vi "Read Items.vi"(8 "error in (no error)":errorcluster, 10 "After (all)":timestamp, 11 "Feed.lvclass in":refnum<class "Feed.lvclass">) -> (0 "error out":errorcluster, 2 "Items":refnum<class "FeedItem.lvclass">[](array[class]), 3 "Feed.lvclass out":refnum<class "Feed.lvclass">)   [LabVIEW 2020, in "Feed.lvclass"]
uses:
  <vilib>/NI_RSS/Feed/Feed.lvclass
  <vilib>/NI_RSS/FeedItem/FeedItem.lvclass
  <vilib>/NI_RSS/Feed/Feed.lvclass/Feed.ctl
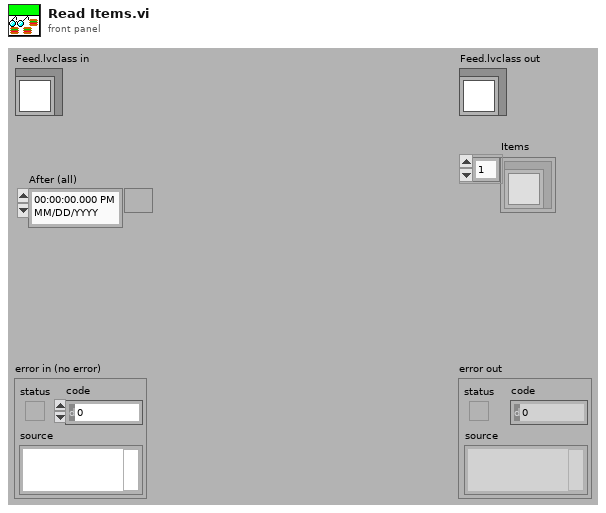
[diagram p1: front panel]
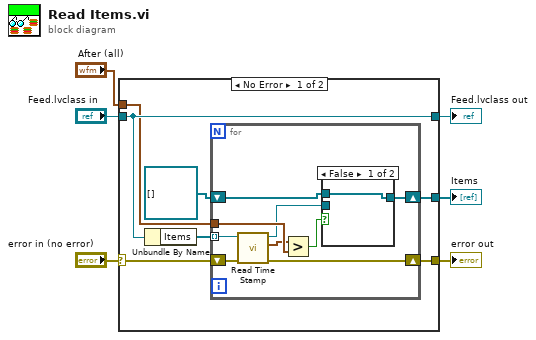
[diagram p0: block diagram]
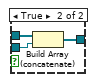
[diagram p2: hidden frame]
diagram:
  n1 = case shown="No Error" "error in (no error)" {
    selector: "error in (no error)" -> [w10 w27]
    tunnel: [w9 w27] -> w5
    tunnel: [w13 w28] -> w3
    tunnel: "Feed.lvclass in" -> [w13 w28]
    tunnel: [w7 _] -> w2
    tunnel: "After (all)" -> [w11 _]
    frame No Error {
      n2 = Unbundle By Name(w13) -> ("Items"=w12:refnum<class "FeedItem.lvclass">[])
      n3 = for {
        tunnel: w12 -> [w21] mode=indexing
        shift-right: [w14] -> w7
        shift-left: refnum<class "FeedItem.lvclass">[] [] -> [w16]
        tunnel: w11 -> [w22]
        shift-right: [w18] -> w9
        shift-left: w10 -> [w19]
        n4 = call-dynamic "Read Time Stamp.vi"("error in (no error)"=w19, "FeedItem.lvclass in"=w21) -> ("error out"=w18:errorcluster, "Time Stamp"=w20:timestamp, "FeedItem.lvclass out"=w15:refnum<class "FeedItem.lvclass">)  [unwired: 7 out]
        n5 = Greater?(x=w20, y=w22) -> (0:w17:bool)
        n6 = case shown="False" w17 {
          tunnel: w16 -> [w23 w26]
          tunnel: w15 -> [_ w25]
          tunnel: [w23 w24] -> w14
          frame False {
          }
          frame True {
            n7 = Build Array (concatenate)(w26, w25) -> (w24:refnum<class "FeedItem.lvclass">[])
          }
        }
      }
    }
    frame Error {
    }
  }
  "error out" <- w5
  "Feed.lvclass out" <- w3
  "Items" <- w2
